vi "KickToSkill_v3.vi"(1 "target gap":dbl[](array[numeric]), 4 "kick_z":dbl, 5 "KickTarget":dbl[](array[numeric]), 6 "kick_x":dbl=50.0, 7 "firstCall?":bool, 8 "error in (no error)":errorcluster, 9 "Game":refnum<class "Game.lvclass">, 10 "Robot":refnum<class "Robot.lvclass">, 11 "KickToSkill in":refnum<class "KickToSkill.lvclass">) -> (0 "error out":errorcluster, 2 "Robot out":refnum<class "Robot.lvclass">, 3 "KickToSkill out":refnum<class "KickToSkill.lvclass">)   [LabVIEW 2023, in "KickToSkill.lvclass"]
uses:
  KickToSkill.lvclass
  Robot_class/Robot.lvclass
  C:/Users/lucio/Desktop/roboime/SSL_AI/Object_class/Object.lvclass
  Game_class/Game.lvclass
  KickToSkill_v3_states.ctl
  Game_class/Game.lvclass/Game.ctl
  Parameters_class/Parameters.lvclass/Parameters.ctl
  Ball_class/Ball.lvclass/Ball.ctl
  Object_class/Object.lvclass/Object.ctl
  Robot_class/robotKickToStates.ctl
  Robot_class/Robot.lvclass/Robot.ctl
  Object_class/Read position(x,y).vi
  Robot_class/Write robotKickState.vi
  Game_class/Read NewParameters.vi
  Game_class/Read BallRef.vi
  Game_class/Read Parameters.lvclass.vi
  Parameters_class/Read AttakingOurselves.vi
  Ball_class/Read velocityNorm.vi
  Robot_class/Write dest_x_kick.vi
  Robot_class/Write dest_y_kick.vi
  <vilib>/Analysis/_algsub.llb/Vector Norm.vi
  <vilib>/Analysis/_algsub.llb/Real Vector Norm.vi
  Ball_class/Ball.lvclass
  Parameters_class/Parameters.lvclass
  Utilities_class/Utilities.lvclass
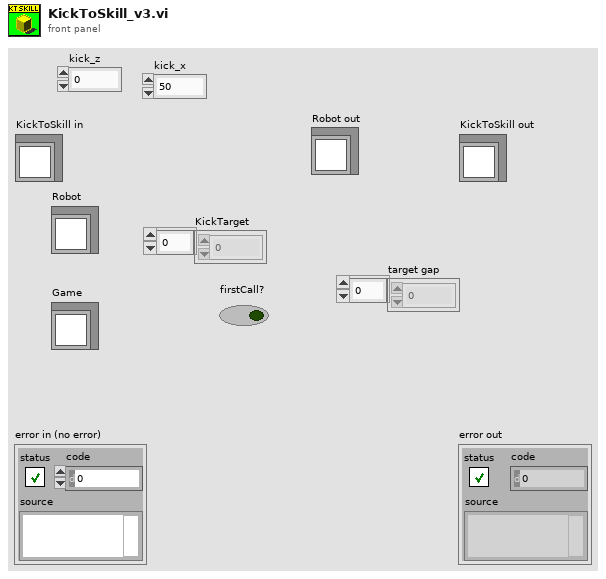
[diagram p1: front panel]
types:
  T1 = typedef "KickToSkill.lvclass/KickToSkill_v3_states.ctl" = enum16{"kick", "align", "turnAntiClockwise", "turnClockwise", "approximate"}
  T2 = typedef "robotKickToStates.ctl" = enum16{"shootFromDirect", "avoidCollideBall", "goToBackBall", "none", "walk", "turn", "turnAntiClockWise", "turnClockwise", "oldKickToShoot", "oldKickToGoToBackBall", "shoot"}
  T3 = typedef "NewParameters.ctl" = cluster{"PenaltyDistance":dbl, "DistanceAttackerToBackBall":dbl, "Division":enum16{"Div B", "Div A"}, "DistanceToAvoidyEnemyRobot":dbl, "BallPlacementDistance":dbl, "DisatanceBehindBallToStealBall":dbl, "MaxDistanceToPositionKickoff":dbl, "BlockEnemyTarget":bool, "MaxStopVAng":dbl, "DistanceMarkerToEnemy":dbl, "IgnoreDribblerContact":bool, "DistanceToBeginEnemyPosession":dbl, "GoToBallWhenEnemyNotMoving":bool, "EnemyDistanceToReduceVelocity":dbl, "TurnOnEnemyDistanceToReduceVelocity":bool, "EnemyDistanceToShootOutBall":dbl, "DefenseKickBall":bool, "MoreKickToGoal? (0-0.3)":dbl, "ChipKickInEnemyField":bool, "ShootOutRobotId":dbl, "FieldLenghtDenominatorInShootOut":dbl, "AdjustPositionInBallPlacement":bool, "PowerGodPass":dbl, "VelocityAbortEnemyPos":dbl, "MaxDistToBeginPass":dbl, "MinDistToBeginPass":dbl, "VelocityInDirects":dbl, "BadDribblerIDs":i32[], "NewKickToDistanceAroundBall":dbl, "PowerAvoidColisionMarker":dbl, "DistanceToAvoidColisionMarker":dbl, "AvoidBallKick":dbl, "DistanceTryKick":dbl, "SuicideKickDIstance":dbl, "AdjustFirstKickDistance":dbl, "AvoidAimLessKick":dbl, "DistanceToAvoidyEnemyShootRobot ":dbl, "NumberOfMarkers":dbl, "PotField":bool, "PIDLateral":bool, "MinDistanceFirstKickX":dbl, "MinDistanceFirstKickY":dbl, "FractionOfDistToTouchGround\nAfterChipKick":dbl, "FractionOfKickxWhen\nComposedWithKickz":dbl, "Style":T4, "MoveInTurnState":bool, "DistFromEnemyToConsider\nMoveInTurnState":dbl, "CascadePID":bool, "TurnAroundParameters":cluster{"Radius":dbl, "Multiplier":dbl, "ChordAngle":dbl}, "SafeDriveVel":dbl, "DistanceToGoToBackBall":dbl, "minDistanceToNotFinish\nEnemyPossession":dbl, "OneTouchShot":cluster{"angleFactor":dbl, "maxAngle":dbl, "Attack":bool, "Defense":bool}, "OpenAngleToGoal":cluster{"minAngle":dbl, "maxAngle":dbl, "minEvaluation":dbl}, "ShotInterception":cluster{"shotSpeed":dbl, "minEnemySpeed":dbl, "maxEnemySpeed":dbl, "minEvaluation":dbl}, "AllyTeamArray":T5[], "maxDefendersNumber":i32, "Zone":cluster{"GuardPositionArray":dbl[][], "ZoneMidField":dbl[], "CenterForwardWidth":dbl}, "MinEvaluationToShoot":dbl, "PassInterception":cluster{"maxPassSpeed":dbl, "minPassSpeed":dbl, "minEnemySpeed":dbl, "chipPassDistance":dbl, "chipPassEvaluation":dbl, "minEvaluation":dbl, "maxEnemySpeed":dbl}, "PassDistance":cluster{"maxDistance":dbl, "minDistance":dbl}, "receiverSpeed":dbl, "maxBallSpeed":dbl, "slackTime":dbl, "Turning radius":dbl, "Turning v_ang":dbl, "AlignError":cluster{"Distance":dbl, "Orientation":dbl, "V_norm(m/s)":dbl, "V_ang (rad/s)":dbl}, "RobotRadius":dbl, "KickerDistance":dbl, "keeper angle  to cover goalpost":dbl}
  T4 = typedef "Style.ctl" = enum16{"Insanity", "Offensive", "Defensive"}
  T5 = typedef "AllyTeam.ctl" = enum16{"Keeper", "Defender", "Attacker"}
  T6 = cluster{"Distance":dbl, "Orientation":dbl, "V_norm(m/s)":dbl, "V_ang (rad/s)":dbl}
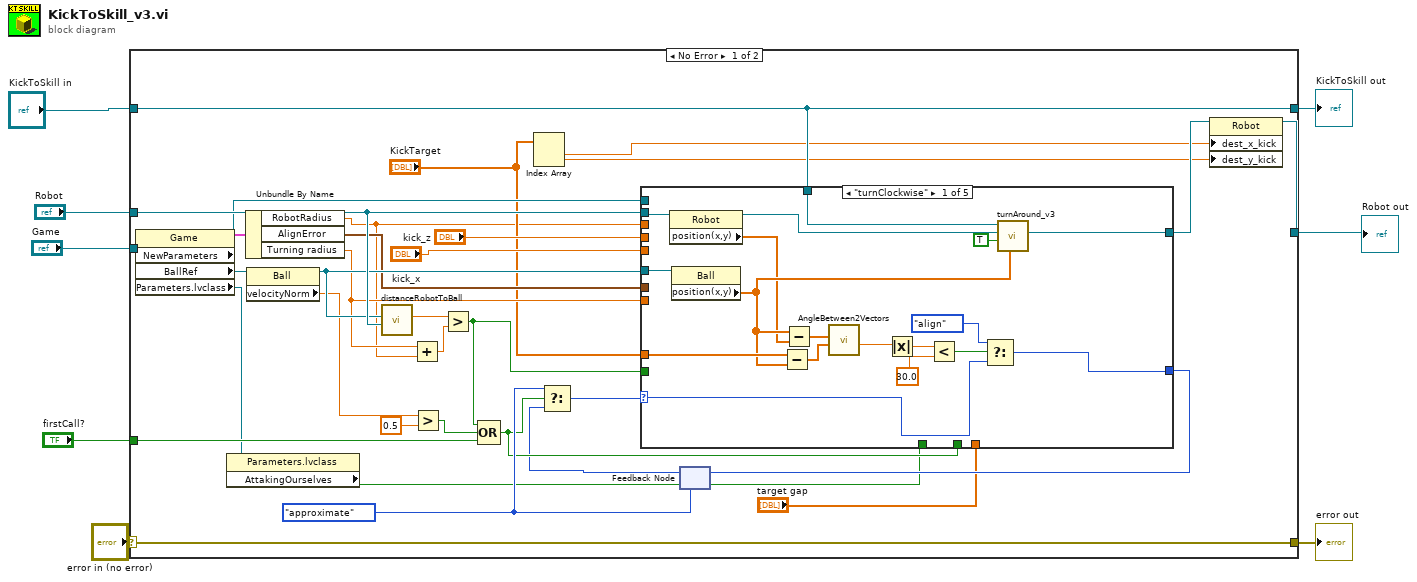
[diagram p0: block diagram]
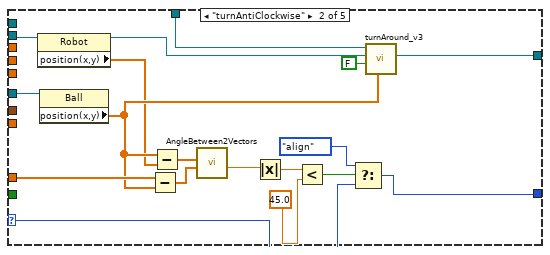
[diagram p2: hidden frame]
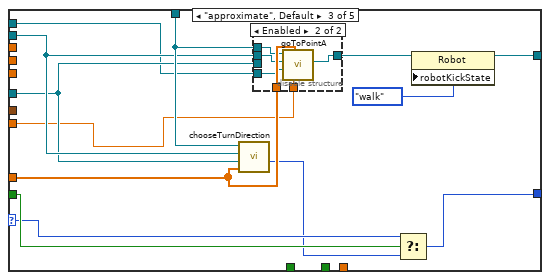
[diagram p3: hidden frame]
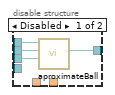
[diagram p4: hidden frame]
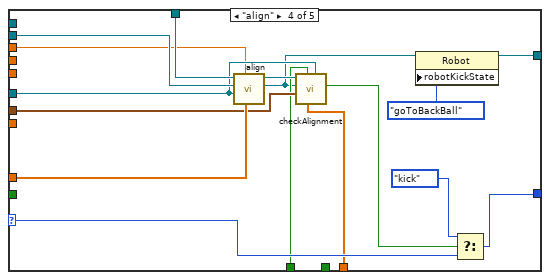
[diagram p5: hidden frame]
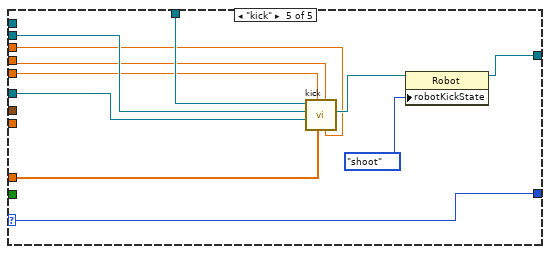
[diagram p6: hidden frame]
diagram:
  n1 = case shown="No Error" "error in (no error)" {
    selector: "error in (no error)" -> [w41 w130]
    tunnel: [w41 w130] -> w7
    tunnel: [w28 w129] -> w5
    tunnel: "KickToSkill in" -> [w28 w129]
    tunnel: "Robot" -> [w39 w128]
    tunnel: "Game" -> [w40 _]
    tunnel: [w23 w128] -> w2
    tunnel: "firstCall?" -> [w16 _]
    frame No Error {
      w37 = KickToSkill_v3_states."approximate" ("States")
      n2 = property class="Game"(reference=w40) -> (reference out=w30:refnum<class "Game.lvclass">, "NewParameters"=w32:T3, "BallRef"=w36:refnum<class "Ball.lvclass">, "Parameters.lvclass"=w13:refnum<class "Parameters.lvclass">)  [unwired: 1 in, 1 out]
      n3 = property class="Parameters.lvclass"(reference=w13) -> ("AttakingOurselves"=w12:bool)  [unwired: 1 in, 2 out]
      n4 = Unbundle By Name(w32) -> ("RobotRadius"=w10:dbl, "AlignError"=w29:T6, "Turning radius"=w31:dbl)
      n5 = property class="Ball"(reference=w36) -> (reference out=w35:refnum<class "Ball.lvclass">, "velocityNorm"=w33:dbl)  [unwired: 1 in, 1 out]
      n6 = call "distanceRobotToBall.vi"("Robot"=w39, "Ball"=w35) -> ("Distance Robot To Ball"=w18:dbl)  [unwired: 7 in, 2 out]
      n7 = Add(x=w31, y=w10) -> (x+y=w19:dbl)
      n8 = Greater?(x=w33, y=0.5) -> (0:w34:bool)
      n9 = Greater?(x=w18, y=w19) -> (0:w17:bool)
      n10 = Compound Arithmetic op=OR(w17, w34, w16) -> (w14:bool)
      n11 = Index Array(array="KickTarget") -> (element #1=w21:dbl, element #2=w20:dbl)  [unwired: 2 in]
      n12 = feedback #1(w37) -> (w11:T1)
      n13 = Select(t=w37, s=w14, f=w11) -> (s? t:f=w9:T1)
      n14 = case shown="\"turnClockwise\"" w9 {
        selector: w9 -> [w44 w63 w82 w114 w127]
        tunnel: w39 -> [w53 w71 w88 w116 w124]
        tunnel: w28 -> [w59 w77 w89 w111 w126]
        tunnel: w35 -> [w57 w75 w87 w106 w125]
        tunnel: [w58 w76 w79 w103 w118] -> w24
        tunnel: [w45 w60 w90 w113 w127] -> w38
        tunnel: "KickTarget" -> [w50 w68 w86 w115 w123]
        tunnel: "kick_x" -> [_ _ _ _ w122]
        tunnel: "kick_z" -> [_ _ _ _ w121]
        tunnel: w31 -> [_ _ w85 _ _]
        tunnel: w30 -> [_ _ w84 _ _]
        tunnel: w29 -> [_ _ _ w109 _]
        tunnel: w17 -> [_ _ w83 _ _]
        tunnel: w14 -> [_ _ _ _ _]
        tunnel: "target gap" -> [_ _ _ w108 _]
        tunnel: w12 -> [_ _ _ w107 _]
        tunnel: w10 -> [_ _ _ w101 w117]
        frame "turnClockwise" {
          n15 = property class="Robot"(reference=w53) -> (reference out=w52:refnum<class "Robot.lvclass">, "position(x,y)"=w47:dbl[])  [unwired: 1 in, 1 out]
          n16 = property class="Ball"(reference=w57) -> ("position(x,y)"=w49:dbl[])  [unwired: 1 in, 2 out]
          n17 = Subtract(x=w50, y=w49) -> (x-y=w48:dbl[])
          n18 = Subtract(x=w49, y=w47) -> (x-y=w51:dbl[])
          n19 = call "AngleBetween2Vectors.vi"("Array 1"=w48, "Array 2"=w51) -> ("angleInDegrees"=w56:dbl)  [unwired: 6 in, 3 out]
          n20 = Absolute Value(x=w56) -> (abs(x)=w55:dbl)
          n21 = Less?(x=w55, y=30.0) -> (x < y?=w46:bool)
          n22 = Select(t=KickToSkill_v3_states."align", s=w46, f=w44) -> (s? t:f=w45:T1)
          n23 = call "turnAround_v3.vi"("Center"=w49, "clockwise?"=TRUE, "Robot"=w52, "KickToSkill in"=w59) -> ("Robot out"=w58:refnum<class "Robot.lvclass">)  [unwired: 5 in, 2 out]
        }
        frame "turnAntiClockwise" {
          n24 = property class="Robot"(reference=w71) -> (reference out=w70:refnum<class "Robot.lvclass">, "position(x,y)"=w65:dbl[])  [unwired: 1 in, 1 out]
          n25 = property class="Ball"(reference=w75) -> ("position(x,y)"=w67:dbl[])  [unwired: 1 in, 2 out]
          n26 = Subtract(x=w68, y=w67) -> (x-y=w66:dbl[])
          n27 = Subtract(x=w67, y=w65) -> (x-y=w69:dbl[])
          n28 = call "AngleBetween2Vectors.vi"("Array 1"=w66, "Array 2"=w69) -> ("angleInDegrees"=w74:dbl)  [unwired: 6 in, 3 out]
          n29 = Absolute Value(x=w74) -> (abs(x)=w73:dbl)
          n30 = Less?(x=w73, y=45.0) -> (x < y?=w64:bool)
          n31 = Select(t=KickToSkill_v3_states."align", s=w64, f=w63) -> (s? t:f=w60:T1)
          n32 = call "turnAround_v3.vi"("Center"=w67, "clockwise?"=FALSE, "Robot"=w70, "KickToSkill in"=w77) -> ("Robot out"=w76:refnum<class "Robot.lvclass">)  [unwired: 5 in, 2 out]
        }
        frame "approximate", Default {
          n33 = call "chooseTurnDirection.vi"("KickTarget"=w86, "Ball"=w87, "Robot"=w88, "KickToSkill in"=w89) -> ("state"=w81:T1)  [unwired: 5 in, 2 out]
          n34 = disable-structure shown="Enabled" {
            disable-tunnel: [w94 w98] -> w80
            disable-tunnel: w89 -> [w93 w97]
            disable-tunnel: w88 -> [w92 w96]
            disable-tunnel: w87 -> [w91 _]
            disable-tunnel: w86 -> [_ w100]
            disable-tunnel: w85 -> [_ w99]
            disable-tunnel: w84 -> [_ w95]
            frame Disabled {
              n35 = call "aproximateBall.vi"("Ball"=w91, "Robot"=w92, "KickToSkill in"=w93) -> ("Robot out"=w94:refnum<class "Robot.lvclass">)  [unwired: 6 in, 2 out]
            }
            frame Enabled {
              n36 = call "goToPointA.vi"("Raio"=w99, "Target"=w100, "Game"=w95, "Robot in"=w96, "KickToSkill in"=w97) -> ("Robot out"=w98:refnum<class "Robot.lvclass">)  [unwired: 4 in, 2 out]
            }
          }
          n37 = Select(t=w82, s=w83, f=w81) -> (s? t:f=w90:T1)
          n38 = property class="Robot"(reference=w80, "robotKickState"=robotKickToStates."walk") -> (reference out=w79:refnum<class "Robot.lvclass">)  [unwired: 1 in, 1 out]
        }
        frame "align" {
          n39 = call "align.vi"("KickTarget"=w115, "RobotRadius"=w101, "Ball"=w106, "Robot"=w116, "KickToSkill in"=w111) -> ("Robot out"=w104:refnum<class "Robot.lvclass">, "KickToSkill out"=w110:refnum<class "KickToSkill.lvclass">)  [unwired: 4 in, 1 out]
          n40 = call "checkAlignment.vi"("Ball"=w106, "target gap"=w108, "attacking ourselves"=w107, "AlignError"=w109, "Robot"=w104, "KickToSkill in"=w110) -> ("Aligned"=w105:bool)  [unwired: 3 in, 2 out]
          n41 = property class="Robot"(reference=w104, "robotKickState"=robotKickToStates."goToBackBall") -> (reference out=w103:refnum<class "Robot.lvclass">)  [unwired: 1 in, 1 out]
          n42 = Select(t=KickToSkill_v3_states."kick", s=w105, f=w114) -> (s? t:f=w113:T1)
        }
        frame "kick" {
          n43 = call "kick.vi"("robot radius"=w117, "kick_z"=w121, "KickTarget"=w123, "kick_x"=w122, "Ball"=w125, "Robot"=w124, "KickToSkill in"=w126) -> ("Robot out"=w119:refnum<class "Robot.lvclass">)  [unwired: 2 in, 2 out]
          n44 = property class="Robot"(reference=w119, "robotKickState"=robotKickToStates."shoot") -> (reference out=w118:refnum<class "Robot.lvclass">)  [unwired: 1 in, 1 out]
        }
      }
      n45 = feedback-in #1(w38) -> ()
      n46 = property class="Robot"(reference=w24, "dest_x_kick"=w21, "dest_y_kick"=w20) -> (reference out=w23:refnum<class "Robot.lvclass">)  [unwired: 1 in, 1 out]
    }
    frame Error {
    }
  }
  "error out" <- w7
  "KickToSkill out" <- w5
  "Robot out" <- w2
